vi "Quaternion2Axis Angle.vi"(8 "error in (no error)":errorcluster, 11 "q_array":sgl[](array[numeric])=[0.0, 0.0, 0.0, 0.0]) -> (0 "error out":errorcluster, 2 "angle":sgl, 3 "axis":sgl[](array[numeric]))   [LabVIEW 2021, in "QuaternionLibrary.lvlib"]
doc: "extern \"C\" QUATERNIONLIBRARY_API void Quaternion2AxisAngle(float q_array[4], float axis[3], float* angle);"
uses:
  <userlib>/QuaternionLibrary/QuaternionLibrary.lvlib
  <userlib>/QuaternionLibrary/QuaternionLibrary.dll
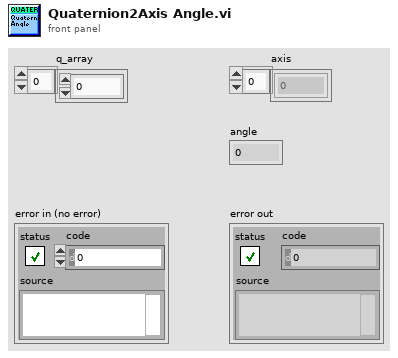
[diagram p1: front panel]
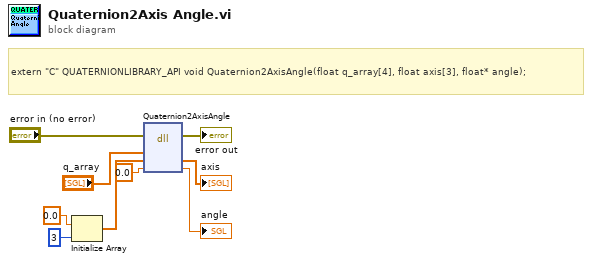
[diagram p0: block diagram]
diagram:
  # "extern \"C\" QUATERNIONLIBRARY_API void Quaternion2AxisAngle(float q_array[4], float axis[3], float* angle);"
  n1 = Initialize Array(sgl 0.0 ("element"), 3 ("dimension size")) -> (w8:sgl[])
  n2 = dll-call lib="C:/Program Files/National Instruments/LabVIEW 2021/user.lib/QuaternionLibrary/QuaternionLibrary.*" fn="Quaternion2AxisAngle"(error in="error in (no error)", "q_array"="q_array", "axis"=w8, "angle"=sgl 0.0) -> (error out=→"error out":errorcluster, "axis"=→"axis":sgl[], "angle"=→"angle":sgl)  [unwired: 4 in, 1 out]
